vi "Core Action.vi"(8 "error in (no error)":errorcluster, 10 "SECS-II Class":refnum<class "SECS-II Class.lvclass">, 11 "12-Upload Alarm Information in":refnum<class "12-Upload Alarm Information.lvclass">) -> (0 "error out":errorcluster, 2 "SECS-II Class Out":refnum<class "SECS-II Class.lvclass">, 3 "12-Upload Alarm Information out":refnum<class "12-Upload Alarm Information.lvclass">)   [LabVIEW 2020, in "SECS Scenarios.lvlib" / "12-Upload Alarm Information.lvclass"]
uses:
  12-Upload Alarm Information.lvclass
  D:/Dropbox/SECS/SECS_GEM v1.1.0/Com/SECS Scenarios/Scenarios Class/Scenarios Class.lvclass
  SECS Communication/SECS-II Class/SECS-II Class.lvclass
  SECS Communication/S5 Message Class/S5 Message Class.lvclass
  D:/Dropbox/SECS/SECS_GEM v1.1.0/Com/SECS Communication/SECS-II Class/SECS-II Class.lvclass
  Scenarios Class/Reply State.ctl
  Scenarios Class/Scenarios Class.lvclass/Scenarios Class.ctl
  Scenarios Class/Write Reply State.vi
  Scenarios Class/Read HSMS Class.vi
  SECS Communication/SECS Data Class/Get ALID Data.vi
  SECS Communication/SECS Data Class/Get All ALID Data.vi
  SECS Communication/HSMS Class/HSMS Class.lvclass
  SECS Communication/SECS Data Class/SECS Data Class.lvclass
  Scenarios Class/Scenarios Class.lvclass
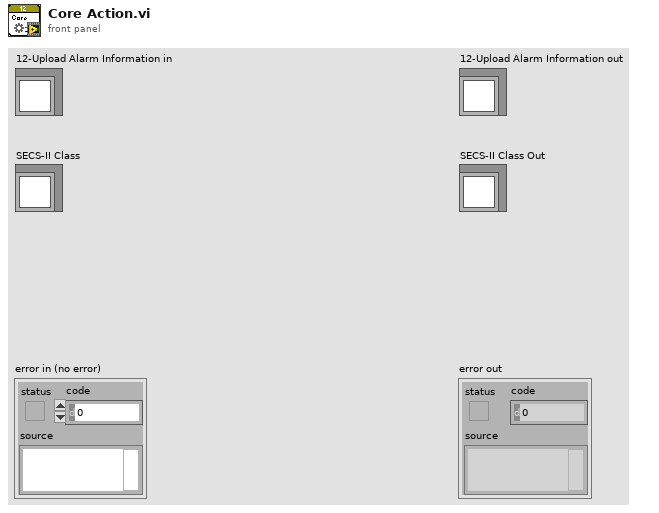
[diagram p1: front panel]
types:
  T1 = typedef "SECS Scenarios.lvlib/Scenarios Class.lvclass/Reply State.ctl" = enum16{"OK", "Illegal Data", "Unknown Stream", "Unknown Function", "Off-Line", "T3 Timeout", "Inner-Timeout"}
  T2 = cluster{"ALCD(Bit8)":bool, "ALID":u32, "ALTX":string}
  T3 = typedef "SECS Communication.lvlib/SECS Data Class.lvclass/ALID Data.ctl" = cluster{"Enable":bool, "ALID":u32, "Name":string, "Description":string, "Source":string, "Status":enum16{"Null", "Normal", "Abnormal", "Warning"}}
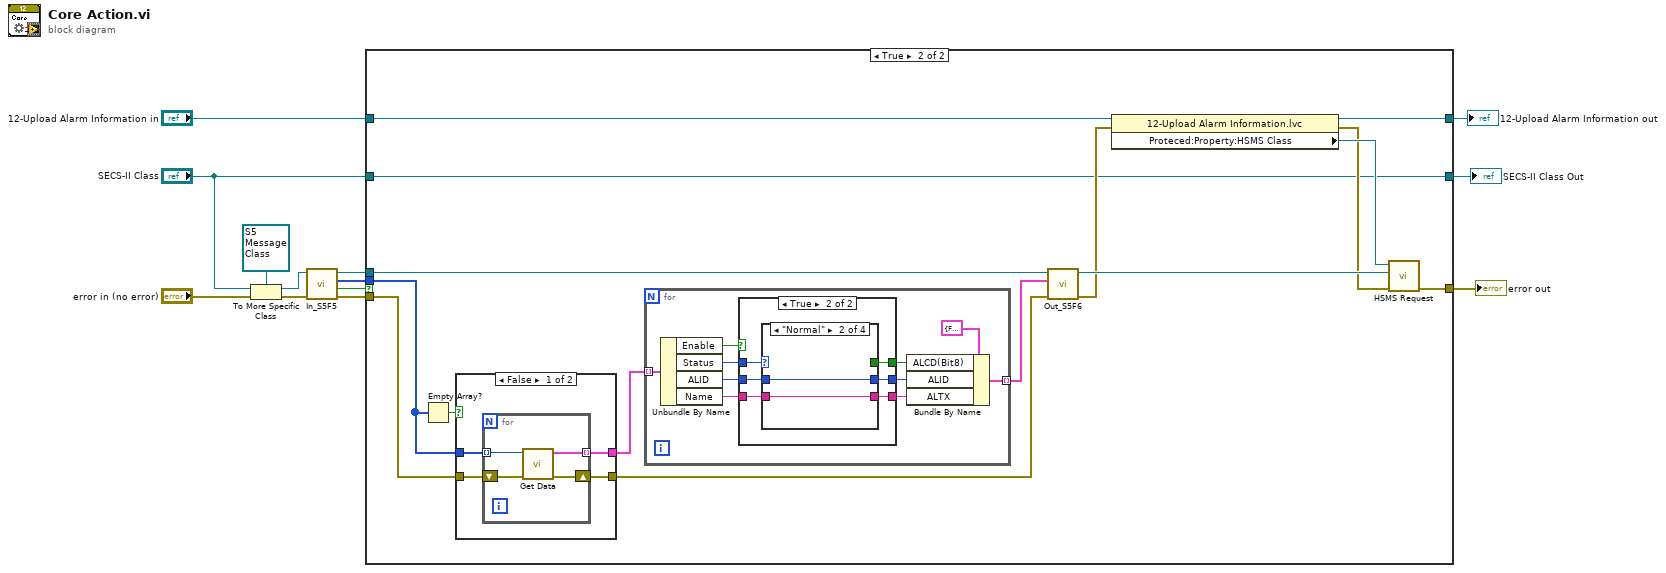
[diagram p0: block diagram]
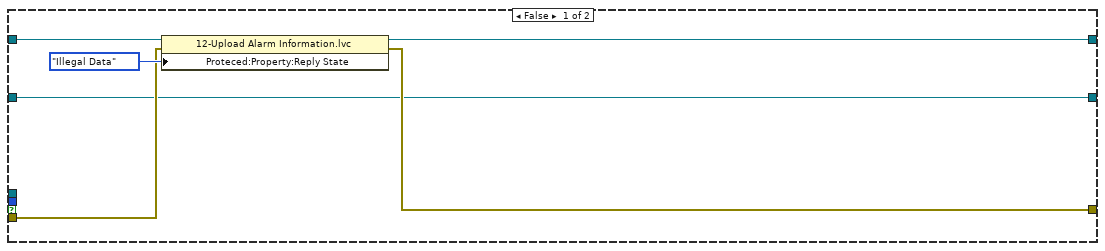
[diagram p2: hidden frame]
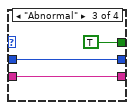
[diagram p5: hidden frame]
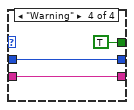
[diagram p6: hidden frame]
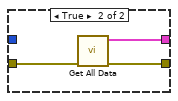
[diagram p7: hidden frame]
diagram:
  n1 = To More Specific Class(target class=refnum<class "S5 Message Class.lvclass"> refnum ("SECS Communication.lvlib:S5 Message Class.lvclass"), reference="SECS-II Class", error in="error in (no error)") -> (specific class reference=w10:refnum<class "S5 Message Class.lvclass">, error out=w11:errorcluster)
  n2 = call "In_S5F5.vi"("error in (no error)"=w11, "S5 Message Class in"=w10) -> ("error out"=w8:errorcluster, "OK?"=w3:bool, "ALIDVECTOR"=w7:u32[], "S5 Message Class out"=w6:refnum<class "S5 Message Class.lvclass">)  [unwired: 6 in]
  n3 = case shown="True" w3 {
    tunnel: "12-Upload Alarm Information in" -> [w19 w34]
    tunnel: [w18 w33] -> w9
    tunnel: w8 -> [w16 w30]
    tunnel: w7 -> [_ w29]
    tunnel: w6 -> [_ w27]
    tunnel: [w15 w22] -> w5
    tunnel: "SECS-II Class" -> [w14 w21]
    tunnel: [w14 w21] -> w1
    frame False {
      n4 = property class="12-Upload Alarm Information.lvc"(reference=w19, error in=w16, "Proteced:Property:Reply State"=Reply_State."Illegal Data" ("Reply State")) -> (reference out=w18:refnum<class "12-Upload Alarm Information.lvclass">, error out=w15:errorcluster)
    }
    frame True {
      n5 = Empty Array?(array=w29) -> (empty?=w31:bool)
      n6 = case shown="False" w31 {
        tunnel: [w66 w71] -> w26
        tunnel: w30 -> [w65 w73]
        tunnel: w29 -> [w64 _]
        tunnel: [w63 w72] -> w28
        frame False {
          n7 = for {
            shift-right: [w70] -> w66
            shift-left: w65 -> [w69]
            tunnel: w64 -> [w68] mode=indexing
            tunnel: [w67] -> w63 mode=indexing
            n8 = call-poly "Get Data.vi"("error in"=w69, "ALID"=w68) -> ("error out"=w70:errorcluster, "ALID Data"=w67:T3)  [unwired: 7 in, 1 out]
          }
        }
        frame True {
          n9 = call-poly "Get All Data.vi"("error in (no error)"=w73) -> ("error out"=w71:errorcluster, "ALID Data"=w72:T3[])  [unwired: 9 in]
        }
      }
      n10 = for {
        tunnel: w28 -> [w39] mode=indexing
        tunnel: [w44] -> w20 mode=indexing
        n11 = Unbundle By Name(w39) -> ("Enable"=w43:bool, "Status"=w42:enum16{"Null", "Normal", "Abnormal", "Warning"}, "ALID"=w41:u32, "Name"=w40:string)
        n12 = case shown="True" w43 {
          tunnel: w42 -> [_ w52]
          tunnel: w41 -> [w46 w51]
          tunnel: w40 -> [w45 w50]
          tunnel: [w45 w49] -> w35
          tunnel: [w46 w48] -> w36
          tunnel: [_ w47] -> w37
          frame False {
          }
          frame True {
            n13 = case shown="\"Normal\"" w52 {
              tunnel: w51 -> [w54 w55 w58 w61]
              tunnel: w50 -> [w53 w56 w59 w62]
              tunnel: [w53 w56 w59 w62] -> w49
              tunnel: [w54 w55 w58 w61] -> w48
              tunnel: [_ _ TRUE TRUE] -> w47
              frame "Null", Default {
              }
              frame "Normal" {
              }
              frame "Abnormal" {
              }
              frame "Warning" {
              }
            }
          }
        }
        n14 = Bundle By Name(cluster=T2 {"ALCD(Bit8)"=FALSE, "ALID"=0, "ALTX"=""} ("S5F6"), "ALCD(Bit8)"=w37, "ALID"=w36, "ALTX"=w35) -> (w44:T2)
      }
      n15 = call "Out_S5F6.vi"("error in (no error)"=w26, "S5F6"=w20, "S5 Message Class in"=w27) -> ("error out"=w24:errorcluster, "S5 Message Class out"=w25:refnum<class "S5 Message Class.lvclass">)  [unwired: 7 in]
      n16 = property class="12-Upload Alarm Information.lvc"(reference=w34, error in=w24) -> (reference out=w33:refnum<class "12-Upload Alarm Information.lvclass">, error out=w23:errorcluster, "Proteced:Property:HSMS Class"=w32:refnum<class "HSMS Class.lvclass">)
      n17 = call "HSMS Request.vi"("error in (no error)"=w23, "SECS-II Class In"=w25, "HSMS Class in"=w32) -> ("error out"=w22:errorcluster)  [unwired: 7 in, 1 out]
    }
  }
  "error out" <- w5
  "12-Upload Alarm Information out" <- w9
  "SECS-II Class Out" <- w1
